vi "Unit Test VI.vi"() -> ()   [LabVIEW 2017]
uses:
  DPO4104.lvclass
  PPLs/Oscilloscope/Oscilloscope.lvlibp/Custom Controls/Select Cursor.ctl
  PPLs/Oscilloscope/Oscilloscope.lvlibp/Custom Controls/Volts per Division.ctl
  PPLs/Oscilloscope/Oscilloscope.lvlibp/Custom Controls/Analog Channels.ctl
  PPLs/Oscilloscope/Oscilloscope.lvlibp/Custom Controls/Run Control.ctl
  PPLs/Oscilloscope/Oscilloscope.lvlibp/Oscilloscope.lvclass
  C:/Projects/LabVIEW/PPLs/Oscilloscope/Oscilloscope.lvlibp/Oscilloscope.lvclass
  PPLs/Oscilloscope/Oscilloscope.lvlibp
panel:
  out "Status":bool[](array[boolean])
  in  "Trigger Slope (0: Rising)":u16(ring) items=["Rising", "Falling", "Either"]
  in  "Trigger Level (0.0 V)":dbl format="%#_13g"
  in  "Trigger Source (0: Channel 1)":u16(ring) items=["Channel 1", "Channel 2", "Channel 3", "Channel 4", "AC Line", "Aux", "Digital Channel 0", "Digital Channel 1", "Digital Channel 2", "Digital Channel 3", "Digital Channel 4", "Digital Channel 5", "Digital Channel 6", "Digital Channel 7", "Digital Channel 8", "Digital Channel 9", "Digital Channel 10", "Digital Channel 11", "Digital Channel 12", "Digital Channel 13", "Digital Channel 14", "Digital Channel 15", "RF"]
  in  "Trigger Coupling (0 : DC)":u16(ring) items=["DC", "HF Reject", "LF Reject", "Noise Reject", "AC"]
  in  "Run Control":T1
  in  "Active Channel(s)":T2[](array[typedef])
  in  "Read Channel":T2
  in  "Screen Shot Path":path
  out "Multi-Waveform":waveform(dbl)[](graph)
  in  "Read Channels":T2[](array[typedef])
  out "Waveform":waveform(dbl)(graph)
  in  "Secs/div":dbl
  in  "V/div":T3
  in  "Lock Controls?":bool
  out "Position":dbl format="%.9f"
  in  "Cursor":T4
  out "Auto-Cal Passed ? (T:Yes)":bool
  out "Self-Test Passed? (T:Yes)":bool
  in  "Method":T5(ring)
  out "DPO4104 out":refnum<class "DPO4104.lvclass">
  out "error out":errorcluster
  in  "Resource":refnum<visa-resource-name>
  in  "DPO4104":refnum<class "DPO4104.lvclass">
  in  "error in (no error)":errorcluster
  # "Self-Test"
  # "Read Waveform"
  # "Read Multi-Channel Waveform"
  # "OPC - Operation Complete"
  # "RQC - Request Control"
  # "QYE  - Query Error"
  # "Auto-Calibrate"
  # "DDE - DEvice Error"
  # "EXE - Execution Error"
  # "CME - Command Error"
  # "URQ - User  Request"
  # "Get Cursor Position"
  # "PON - Power On"
  # "Lock Controls"
  # "Manual Scale & Select Active Channels"
  # "Set Edge Trigger"
  # "Run Control"
  # "Save Screen Shot"
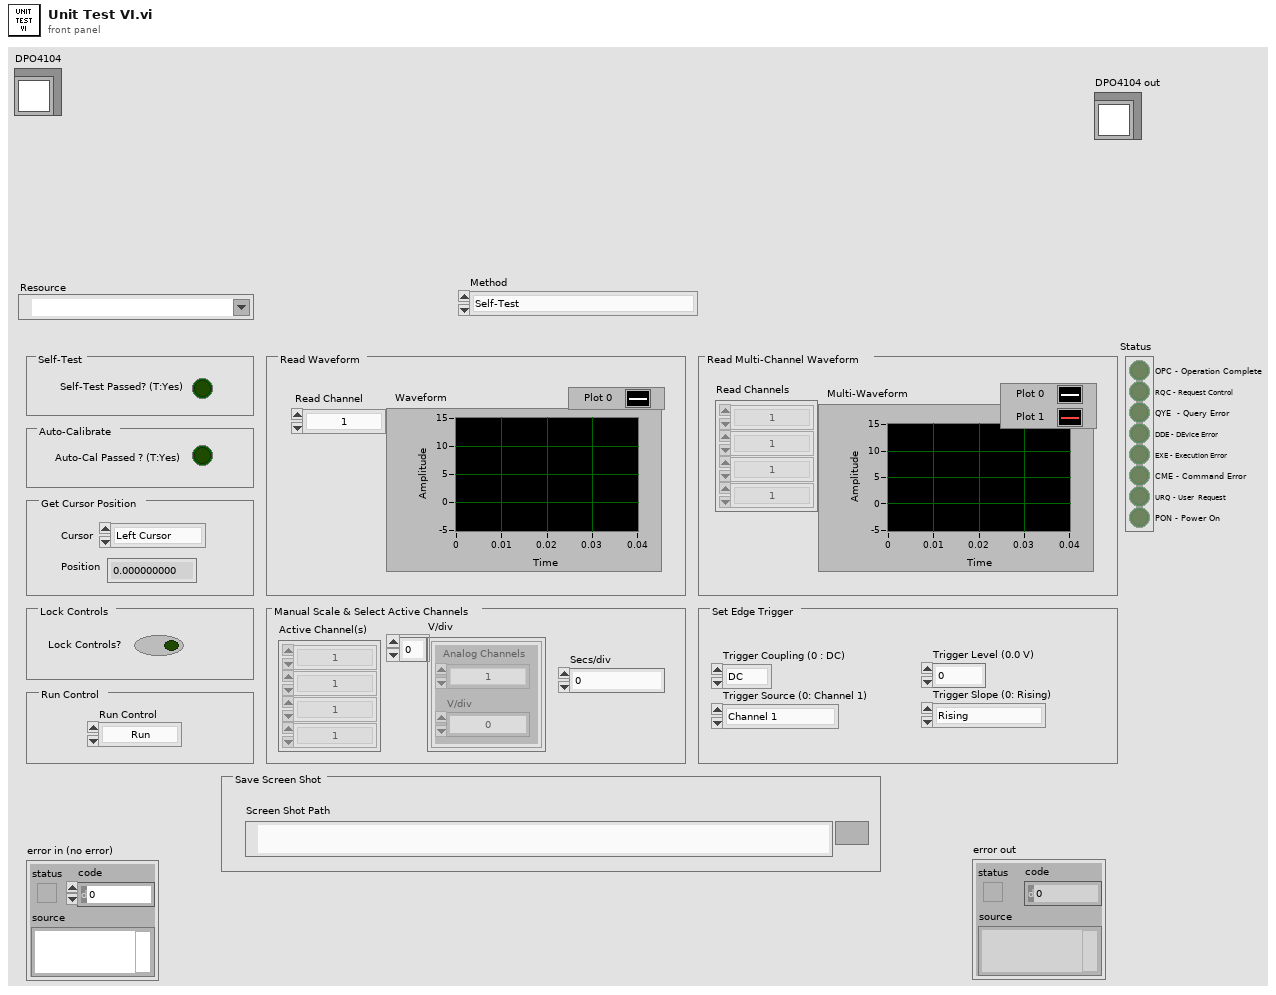
[diagram p1: front panel]
types:
  T1 = typedef "Oscilloscope.lvlibp/Run Control.ctl" = enum16{"Run", "Single", "Stop"}
  T2 = typedef "Oscilloscope.lvlibp/Analog Channels.ctl" = enum16{"1", "2", "3", "4"}
  T3 = typedef "Oscilloscope.lvlibp/Volts per Division.ctl" = cluster{"Analog Channels":T2, "V/div":dbl}[]
  T4 = typedef "Oscilloscope.lvlibp/Select Cursor.ctl" = enum16{"Left Cursor", "Right Cursor", "Top Cursor", "Bottom Cursor"}
  T5 = enum16{"Self-Test", "Auto-Calibrate", "AutoScale", "Get Cursor Position", "Lock Controls", "Manual Scale & Select Active Channels", "Read Waveform", "Read Multi-Channel Waveform", "Save Screenshot", "Select Active Channels", "Set Run Control", "Reset", "Save-Recall Setup", "Set Edge Trigger", "Get Status"}
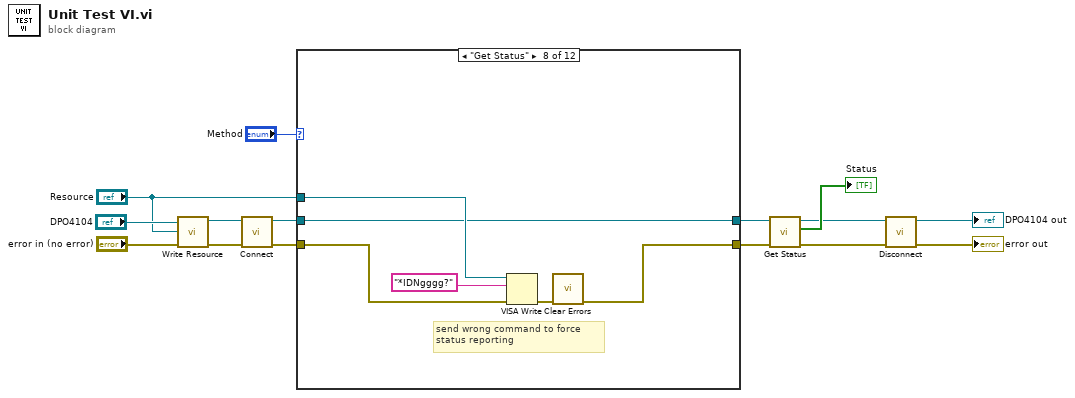
[diagram p0: block diagram]
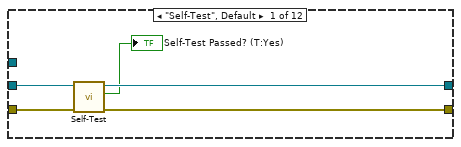
[diagram p2: hidden frame]
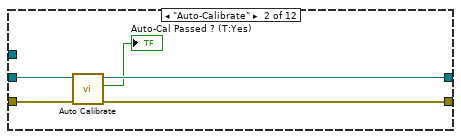
[diagram p3: hidden frame]
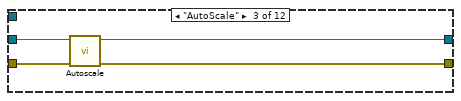
[diagram p4: hidden frame]
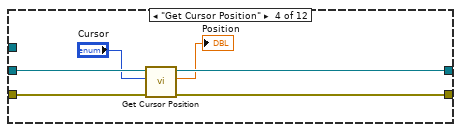
[diagram p5: hidden frame]
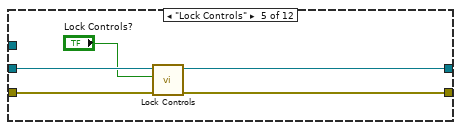
[diagram p6: hidden frame]
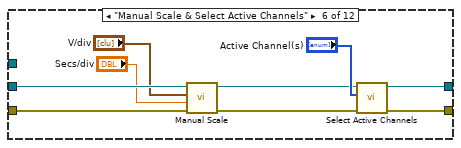
[diagram p7: hidden frame]
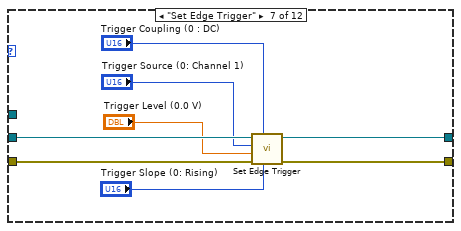
[diagram p8: hidden frame]
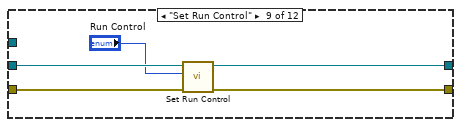
[diagram p9: hidden frame]
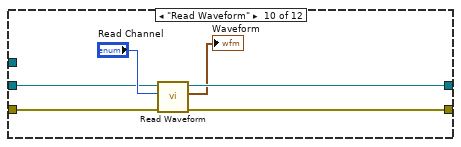
[diagram p10: hidden frame]
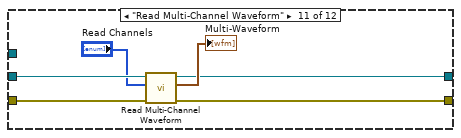
[diagram p11: hidden frame]
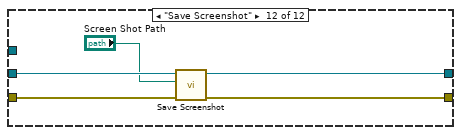
[diagram p12: hidden frame]
diagram:
  n1 = call "Write Resource.vi"("error in (no error)"="error in (no error)", "Resource"="Resource", "Oscilloscope in"="DPO4104") -> ("error out"=w12:errorcluster, "Oscilloscope out"=w13:refnum<class "DPO4104.lvclass">)  [unwired: 7 in]
  n2 = call-dynamic "Connect.vi"("error in (no error)"=w12, "DPO4104 in"=w13) -> ("error out"=w11:errorcluster, "DPO4104 out"=w10:refnum<class "DPO4104.lvclass">)  [unwired: 8 in]
  n3 = case shown="\"Get Status\"" "Method" {
    tunnel: w11 -> [w19 w25 w28 w35 w40 w49 w57 w59 w67 w69 w77 w84]
    tunnel: w10 -> [w20 w24 w29 w34 w39 w48 w56 w58 w68 w70 w78 w85]
    tunnel: [w17 w22 w27 w32 w37 w44 w50 w60 w65 w73 w75 w82] -> w4
    tunnel: [w18 w23 w26 w33 w38 w45 w51 w58 w66 w74 w79 w83] -> w5
    tunnel: "Resource" -> [_ _ _ _ _ _ _ w63 _ _ _ _]
    frame "Self-Test", Default {
      n4 = call-dynamic "Self-Test.vi"("error in (no error)"=w19, "DPO4104 in"=w20) -> ("error out"=w17:errorcluster, "Self-Test Passed? (T:Yes)"=→"Self-Test Passed? (T:Yes)":bool, "DPO4104 out"=w18:refnum<class "DPO4104.lvclass">)  [unwired: 7 in]
    }
    frame "Auto-Calibrate" {
      n5 = call-dynamic "Auto Calibrate.vi"("error in (no error)"=w25, "DPO4104 in"=w24) -> ("error out"=w22:errorcluster, "Cal Passed ? (T:Yes)"=→"Auto-Cal Passed ? (T:Yes)":bool, "DPO4104 out"=w23:refnum<class "DPO4104.lvclass">)  [unwired: 7 in]
    }
    frame "AutoScale" {
      n6 = call-dynamic "Autoscale.vi"("error in (no error)"=w28, "DPO4104 in"=w29) -> ("error out"=w27:errorcluster, "DPO4104 out"=w26:refnum<class "DPO4104.lvclass">)  [unwired: 8 in]
    }
    frame "Get Cursor Position" {
      n7 = call-dynamic "Get Cursor Position.vi"("error in (no error)"=w35, "Cursor"="Cursor", "DPO4104 in"=w34) -> ("error out"=w32:errorcluster, "Position"=→"Position":dbl, "DPO4104 out"=w33:refnum<class "DPO4104.lvclass">)  [unwired: 6 in]
    }
    frame "Lock Controls" {
      n8 = call-dynamic "Lock Controls.vi"("error in (no error)"=w40, "Lock Controls?"="Lock Controls?", "DPO4104 in"=w39) -> ("error out"=w37:errorcluster, "DPO4104 out"=w38:refnum<class "DPO4104.lvclass">)  [unwired: 7 in]
    }
    frame "Manual Scale & Select Active Channels" {
      n9 = call-dynamic "Manual Scale.vi"("error in (no error)"=w49, "Secs/div"="Secs/div", "V/div"="V/div", "DPO4104 in"=w48) -> ("error out"=w41:errorcluster, "DPO4104 out"=w42:refnum<class "DPO4104.lvclass">)  [unwired: 6 in]
      n10 = call-dynamic "Select Active Channels.vi"("error in (no error)"=w41, "Active Channel(s)"="Active Channel(s)", "DPO4104 in"=w42) -> ("error out"=w44:errorcluster, "DPO4104 out"=w45:refnum<class "DPO4104.lvclass">)  [unwired: 7 in]
    }
    frame "Set Edge Trigger" {
      n11 = call-dynamic "Set Edge Trigger.vi"("Trigger Slope (0: Rising)"="Trigger Slope (0: Rising)", "Trigger Coupling (0 : DC)"="Trigger Coupling (0 : DC)", "error in (no error)"=w57, "Trigger Level (0.0 V)"="Trigger Level (0.0 V)", "Analog Channels"="Trigger Source (0: Channel 1)", "DPO4104 in"=w56) -> ("error out"=w50:errorcluster, "DPO4104 out"=w51:refnum<class "DPO4104.lvclass">)  [unwired: 4 in]
    }
    frame "Get Status" {
      # "send wrong command to force \nstatus reporting"
      n12 = VISA Write(VISA resource name=w63, write buffer="*IDNgggg?", error in (no error)=w59) -> (error out=w61:errorcluster)  [unwired: 2 out]
      n13 = call <vilib>:"Clear Errors.vi"("error in (no error)"=w61) -> ("error out"=w60:errorcluster)  [unwired: 5 in, 1 out]
    }
    frame "Set Run Control" {
      n14 = call-dynamic "Set Run Control.vi"("error in (no error)"=w67, "Run Control"="Run Control", "DPO4104 in"=w68) -> ("error out"=w65:errorcluster, "DPO4104 out"=w66:refnum<class "DPO4104.lvclass">)  [unwired: 7 in]
    }
    frame "Read Waveform" {
      n15 = call-dynamic "Read Waveform.vi"("error in (no error)"=w69, "Channel"="Read Channel", "DPO4104 in"=w70) -> ("error out"=w73:errorcluster, "Waveform"=→"Waveform":waveform(dbl), "DPO4104 out"=w74:refnum<class "DPO4104.lvclass">)  [unwired: 6 in]
    }
    frame "Read Multi-Channel Waveform" {
      n16 = call-dynamic "Read Multi-Channel Waveform.vi"("error in (no error)"=w77, "Channels"="Read Channels", "DPO4104 in"=w78) -> ("error out"=w75:errorcluster, "Waveform"=→"Multi-Waveform":waveform(dbl)[], "DPO4104 out"=w79:refnum<class "DPO4104.lvclass">)  [unwired: 6 in]
    }
    frame "Save Screenshot" {
      n17 = call-dynamic "Save Screenshot.vi"("error in (no error)"=w84, "Screen Shot Path"="Screen Shot Path", "DPO4104 in"=w85) -> ("error out"=w82:errorcluster, "DPO4104 out"=w83:refnum<class "DPO4104.lvclass">)  [unwired: 7 in]
    }
  }
  n18 = call-dynamic "Get Status.vi"("error in (no error)"=w4, "DPO4104 in"=w5) -> ("error out"=w2:errorcluster, "Status Array"=→"Status":bool[], "DPO4104 out"=w3:refnum<class "DPO4104.lvclass">)  [unwired: 7 in]
  n19 = call-dynamic "Disconnect.vi"("error in (no error)"=w2, "DPO4104 in"=w3) -> ("error out"=→"error out":errorcluster, "DPO4104 out"=→"DPO4104 out":refnum<class "DPO4104.lvclass">)  [unwired: 8 in]
